vi "FixCodeSpacing2.vi"(11 "Code":string) -> (3 "Cleaned":string)   [LabVIEW 2020]
uses:
  <vilib>/Utility/error.llb/whitespace.ctl
panel:
  out "Unique":i32[](array[numeric])
  out "Indents":i32[](array[numeric])
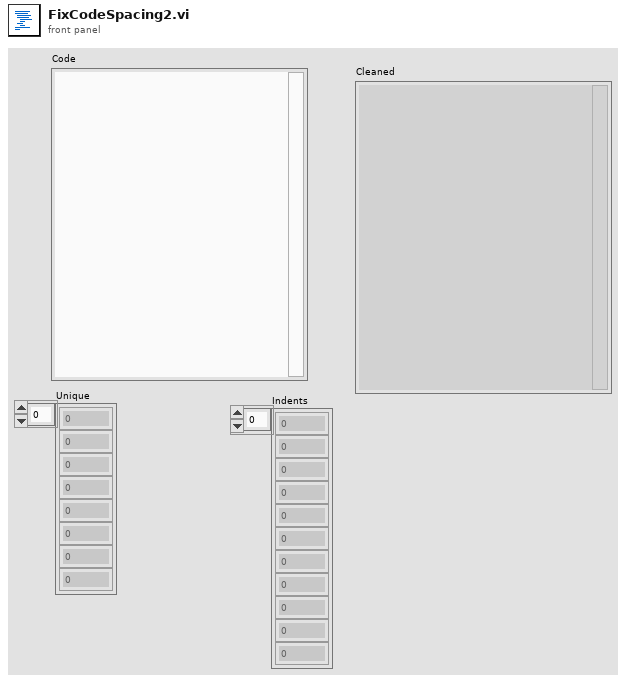
[diagram p1: front panel]
types:
  T1 = typedef "whitespace.ctl" = u16
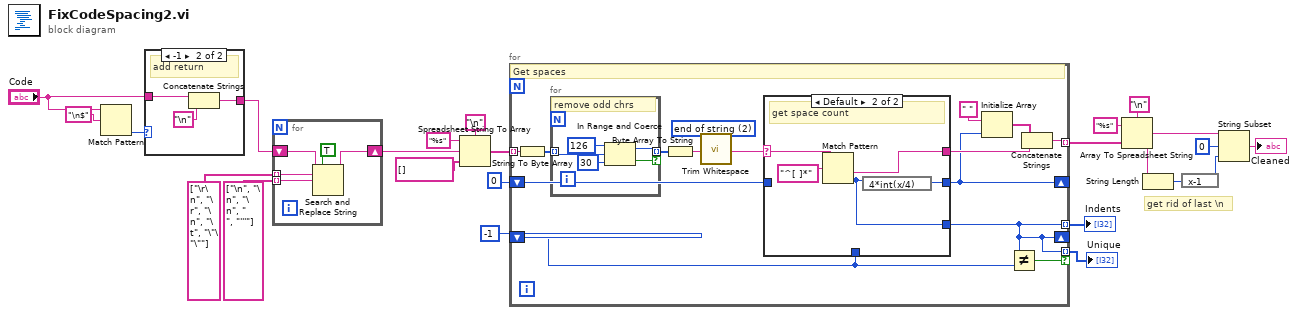
[diagram p0: block diagram]
diagram:
  # "get rid of last \\n"
  n1 = Match Pattern(string="Code", regular expression="\n$" ("search string")) -> (offset past match=w6:i32)  [unwired: 1 in, 3 out]
  n2 = case shown="-1" w6 {
    tunnel: "Code" -> [w24 w27]
    tunnel: [w24 w25] -> w5
    frame Default {
    }
    frame -1 {
      # "add return"
      n3 = Concatenate Strings(w27, "\n" ("search string")) -> (w25:string)
    }
  }
  n4 = for {
    tunnel: string[] ["\r\n", "\r", "\n", "\t", "\"\"\""] -> [w30] mode=indexing
    tunnel: string[] ["\n", "\n", "\n", "    ", "'''"] -> [w29] mode=indexing
    shift-right: [w28] -> w17
    shift-left: w5 -> [w32]
    n5 = Search and Replace String(replace all?=TRUE ("replace all? (F)"), input string=w32, search string=w30, replace string=w29) -> (result string=w28:string)  [unwired: 4 in, 3 out]
  }
  n6 = Spreadsheet String To Array(delimiter (Tab)="\n" ("replace string (\"\")"), format string="%s", spreadsheet string=w17, array type (2D Dbl)=string[] []) -> (array=w4:string[])
  n7 = for {
    tunnel: [w43] -> _ mode=indexing
    tunnel: w4 -> [w43] mode=indexing
    tunnel: [w35] -> w18 mode=indexing
    shift-right: [w35] -> _
    shift-left: -1 ("offset past match") -> [w46]
    tunnel: [w35] -> w15 mode=indexing if=w47
    tunnel: [w39] -> w2 mode=indexing
    shift-right: [w34] -> _
    shift-left: 0 ("offset past match") -> [w33]
    w38 = T1 2 items=["both", "start of string", "end of string"] ("location (both)")
    # "Get spaces"
    n8 = String To Byte Array(string=w43) -> (unsigned byte array=w44:u8[])
    n9 = for {
      tunnel: [w49] -> w45 mode=indexing if=w48
      tunnel: w44 -> [w52] mode=indexing
      # "remove odd chrs"
      n10 = In Range and Coerce(upper limit=u8 126, x=w52, lower limit=u8 30) -> (coerced(x)=w49:u8, In Range?=w48:bool)
    }
    n11 = Byte Array To String(unsigned byte array=w45) -> (string=w37:string)
    n12 = call <vilib>:"Trim Whitespace.vi"("string"=w37, "location (both)"=w38) -> ("trimmed string"=w36:string)
    n13 = case shown="Default" w36 {
      selector: w36 -> [w55 w59]
      tunnel: [w55 w58] -> w40
      tunnel: w46 -> [w54 _]
      tunnel: [w53 w57] -> w34
      tunnel: [w54 w56] -> w35
      tunnel: w33 -> [w53 _]
      frame "" {
        # "blank line"
      }
      frame Default {
        # "get space count"
        n14 = Match Pattern(string=w59, regular expression="^[ ]*") -> (after substring=w58:string, offset past match=w56:i32)  [unwired: 1 in, 2 out]
        n15 = expression code="4*int(x/4)"(w56) -> (w57:i32)
      }
    }
    n16 = Initialize Array(" " ("regular expression"), w34) -> (w41:string[])
    n17 = Not Equal?(x=w35, y=w46) -> (x != y?=w47:bool)
    n18 = Concatenate Strings(w41, w40) -> (w39:string)
  }
  "Indents" <- w18
  "Unique" <- w15
  n19 = Array To Spreadsheet String(delimiter (Tab)="\n" ("replace string (\"\")"), array=w2, 3:"%s" ("format string")) -> (spreadsheet string=w10:string)
  n20 = String Length(string=w10) -> (length=w9:i32)
  n21 = expression code="x-1"(w9) -> (w8:i32)
  n22 = String Subset(string=w10, offset (0)=0, length (rest)=w8) -> (substring=→"Cleaned":string)
